vi "[RT]Intellirupter_Read.vi"() -> ()   [LabVIEW 2016]
uses:
  <vilib>/rvi/interface/nirviOpenFPGA/nirviOpenFPGA.xnode
  <vilib>/rvi/interface/nirviCloseFPGA/nirviCloseFPGA.xnode
  <vilib>/rvi/interface/nirviMethod/nirviMethod.xnode
  <vilib>/rvi/interface/nirviReadWriteControl/nirviReadWriteControl.xnode
  <vilib>/FPGAPlugInAG/Dynamic/niLvFpga_ReadFifo_Dynamic.vi
  <vilib>/rvi/errors/niLvFpgaMergeErrorWithErrorCode.vi
  FPGA Bitfiles/IntelliRupter_FPGATarget_Intelliruptersensor5.lvbitx
  <vilib>/FPGAPlugInAG/cRIO-9039 (Sync)/niLvFpga_Open_cRIO-9039 (Sync).vi
  <vilib>/rvi/interface/common/dynamic/niFpgaDynamicAddResources.vi
  <vilib>/rvi/interface/Simulation/niFpgaSimulationCallBeginRW.vi
  <vilib>/rvi/errors/niLvFpgaAdjustHostInterfaceError.vi
  <vilib>/FPGAPlugInAG/Dynamic/niLvFpga_Close_Dynamic.vi
panel:
  in  "Count(ticks)":u32
  out "Waveform Chart":dbl(graph)
  out "error out":errorcluster
  in  "Relay 2":bool
  in  "Relay 1":bool
  in  "Relay 4":bool
  in  "Relay 3":bool
  in  "Relay 5":bool
  in  "Relay 6":bool
  in  "Relay 8":bool
  in  "Relay 7":bool
  in  "Stop":bool
  out "I8 B":fxp<+/-,26,5>
  out "I8 A":fxp<+/-,26,5>
  out "V8R CA":fxp<+/-,26,5>
  out "V8R BC":fxp<+/-,26,5>
  out "V8R AB":fxp<+/-,26,5>
  out "V5R CA":fxp<+/-,26,5>
  out "V5R BC":fxp<+/-,26,5>
  out "V5R AB":fxp<+/-,26,5>
  out "I5 B":fxp<+/-,26,5>
  out "I5 A":fxp<+/-,26,5>
  out "V5L CA":fxp<+/-,26,5>
  out "V5L BC":fxp<+/-,26,5>
  out "V5L AB":fxp<+/-,26,5>
  out "V4L CA":fxp<+/-,26,5>
  out "V4L BC":fxp<+/-,26,5>
  out "V4L AB":fxp<+/-,26,5>
  out "I4 C":fxp<+/-,26,5>
  out "I4 B":fxp<+/-,26,5>
  out "I4 A":fxp<+/-,26,5>
  out "V4R CA":fxp<+/-,26,5>
  out "V4R BC":fxp<+/-,26,5>
  out "V4R AB":fxp<+/-,26,5>
  out "V2L CA":fxp<+/-,26,5>
  out "V2L BC":fxp<+/-,26,5>
  out "V2L AB":fxp<+/-,26,5>
  out "I2 C":fxp<+/-,26,5>
  out "I5 C":fxp<+/-,26,5>
  out "I2 B":fxp<+/-,26,5>
  out "I2 A":fxp<+/-,26,5>
  out "V2R CA":fxp<+/-,26,5>
  out "V2R BC":fxp<+/-,26,5>
  out "V2R AB":fxp<+/-,26,5>
  out "V7R CA":fxp<+/-,26,5>
  out "V7R BC":fxp<+/-,26,5>
  out "V7R AB":fxp<+/-,26,5>
  out "I8 C":fxp<+/-,26,5>
  out "V8L CA":fxp<+/-,26,5>
  out "V8L BC":fxp<+/-,26,5>
  out "V8L AB":fxp<+/-,26,5>
  out "I7 C":fxp<+/-,26,5>
  out "I7 B":fxp<+/-,26,5>
  out "I7 A":fxp<+/-,26,5>
  out "V7L CA":fxp<+/-,26,5>
  out "V7L BC":fxp<+/-,26,5>
  out "V7L AB":fxp<+/-,26,5>
  out "V6R CA":fxp<+/-,26,5>
  out "V6R BC":fxp<+/-,26,5>
  out "V6R AB":fxp<+/-,26,5>
  out "I6 C":fxp<+/-,26,5>
  out "I6 B":fxp<+/-,26,5>
  out "I6 A":fxp<+/-,26,5>
  out "V6L CA":fxp<+/-,26,5>
  out "V6L BC":fxp<+/-,26,5>
  out "V6L AB":fxp<+/-,26,5>
  out "V3L CA":fxp<+/-,26,5>
  out "V3L BC":fxp<+/-,26,5>
  out "V3L AB":fxp<+/-,26,5>
  out "I3 C":fxp<+/-,26,5>
  out "I3 B":fxp<+/-,26,5>
  out "I3 A":fxp<+/-,26,5>
  out "V3R CA":fxp<+/-,26,5>
  out "V3R BC":fxp<+/-,26,5>
  out "V3R AB":fxp<+/-,26,5>
  out "V1L CA":fxp<+/-,26,5>
  out "V1L BC":fxp<+/-,26,5>
  out "V1L AB":fxp<+/-,26,5>
  out "I1 C":fxp<+/-,26,5>
  out "I1 B":fxp<+/-,26,5>
  out "I1 A":fxp<+/-,26,5>
  out "V1R CA":fxp<+/-,12,5>
  out "V1R BC":fxp<+/-,26,5>
  out "V1R AB":fxp<+/-,26,5>
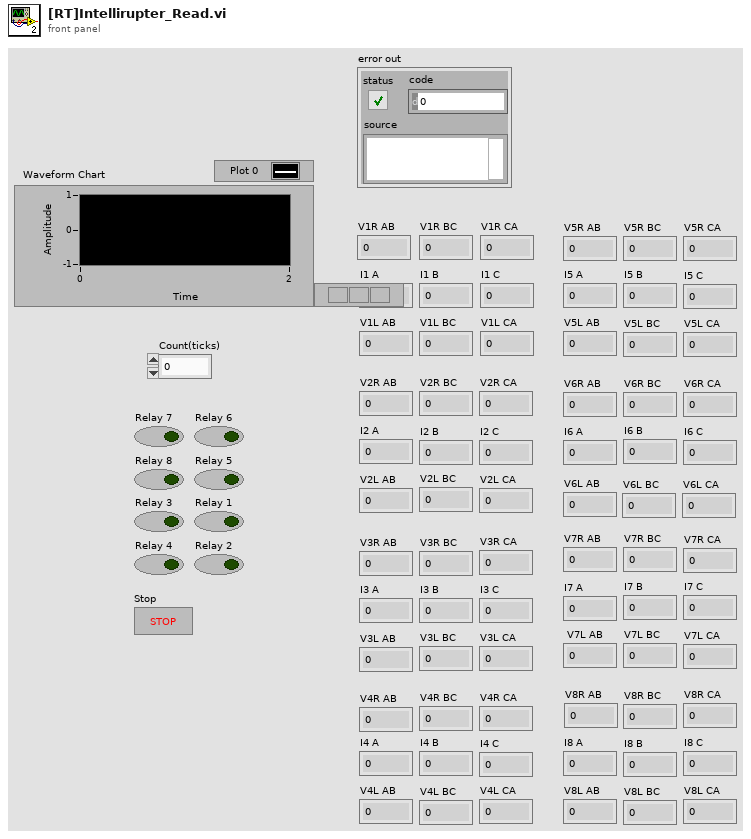
[diagram p1: front panel]
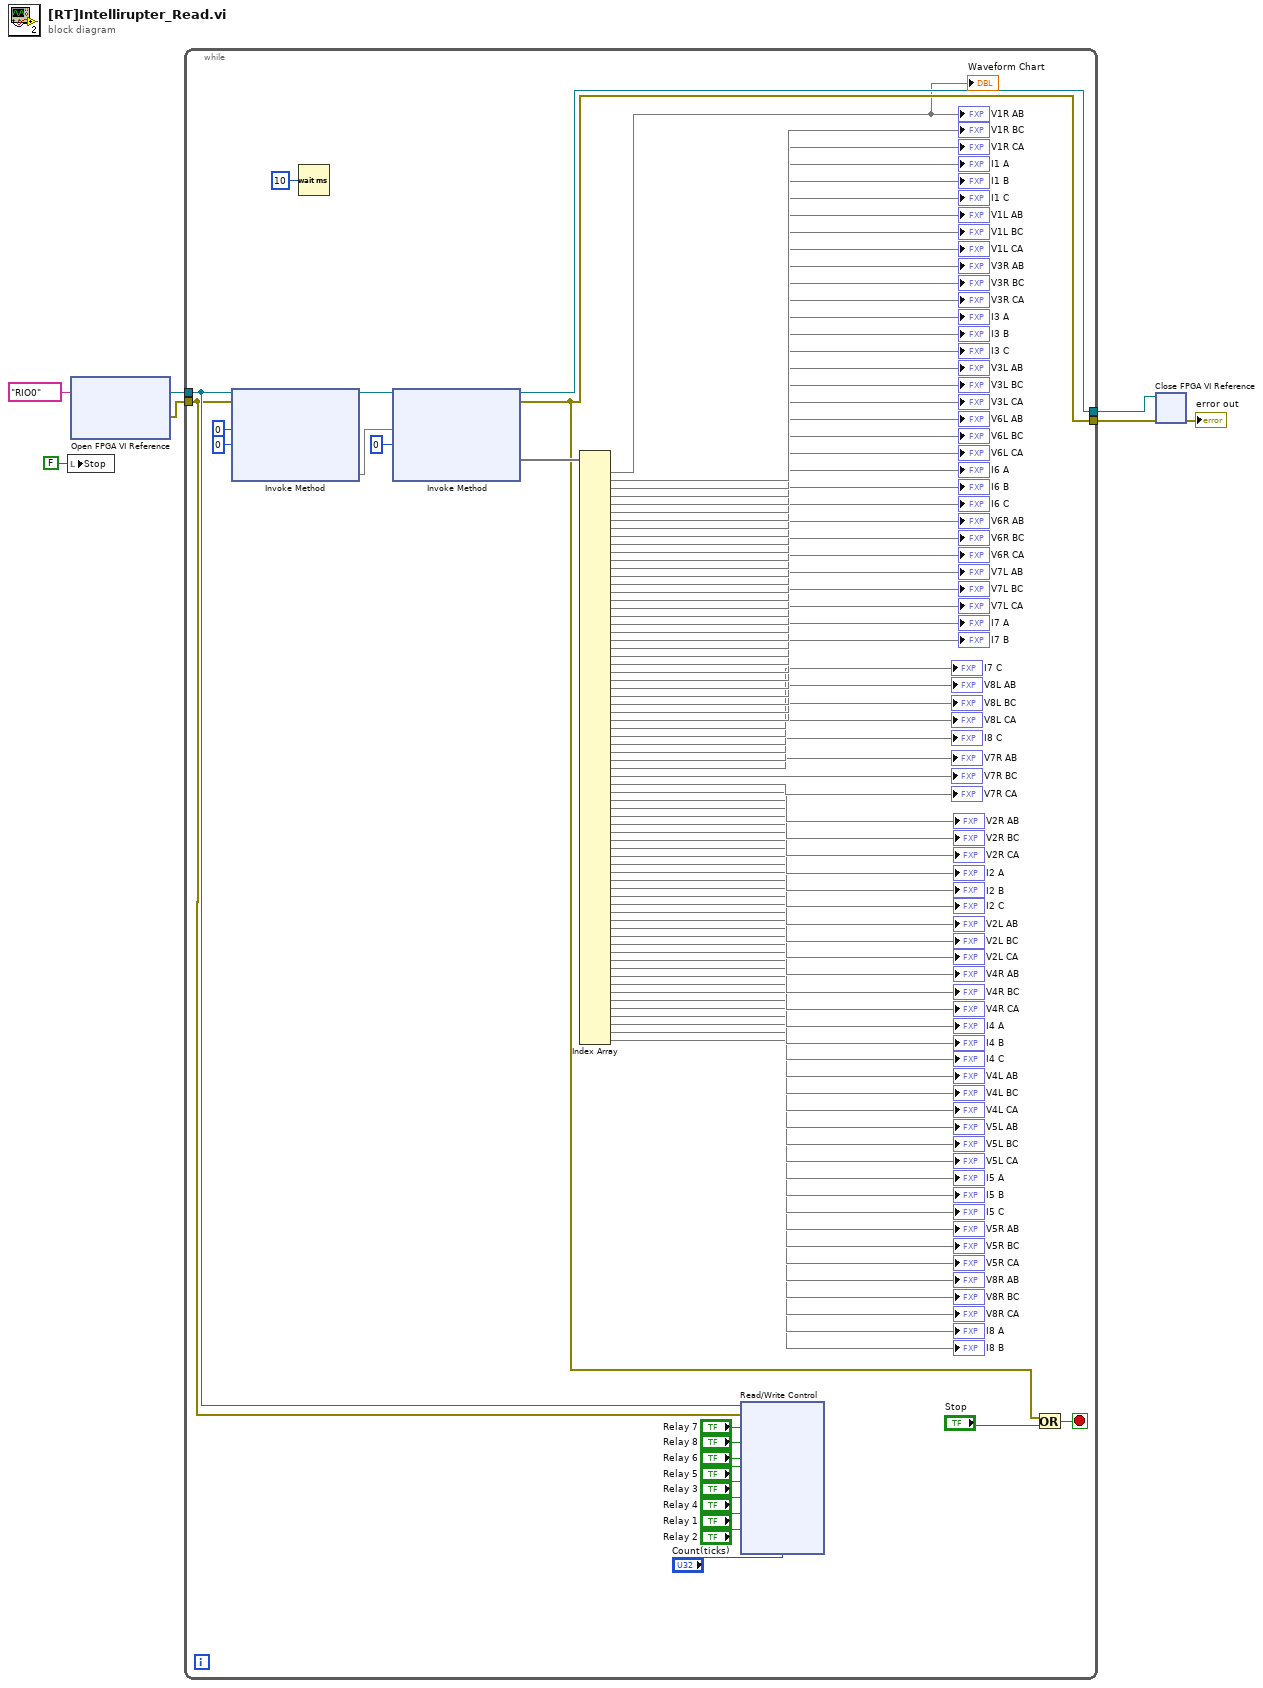
[diagram p0: block diagram]
diagram:
  n1 = local write "Stop"(FALSE ("Stop")) -> ()
  n2 = xnode "Open FPGA VI Reference"("resource name"=tag "RIO0") -> ("FPGA VI Reference Out"=w7:refnum<k20>, "error out"=w6:errorcluster)  [unwired: 1 in]
  n3 = while {
    tunnel: w7 -> [w25]
    tunnel: w6 -> [w24]
    tunnel: [w14] -> w5
    tunnel: [w10] -> w4
    stop <- w30 stop-if-true
    n4 = xnode "Invoke Method"("FPGA VI Reference In"=w25, "error in"=w24, "Number of Elements"=u32 0, "Timeout (ms)"=0) -> ("FPGA VI Reference Out"=w28:refnum<k20>, "Elements Remaining"=w12)  [unwired: 2 out]
    n5 = Wait (ms)(milliseconds to wait=u32 10) -> ()  [unwired: 1 out]
    n6 = xnode "Invoke Method"("FPGA VI Reference In"=w28, "Number of Elements"=w12, "Timeout (ms)"=0) -> ("FPGA VI Reference Out"=w14:refnum<k20>, "error out"=w10:errorcluster, "Data"=w11:void[])  [unwired: 1 in, 1 out]
    n7 = Index Array(array=w11) -> (element #1=→"V1R AB" →"Waveform Chart", element #2=→"V1R BC", element #3=→"V1R CA", element #4=→"I1 A", element #5=→"I1 B", element #6=→"I1 C", element #7=→"V1L AB", element #8=→"V1L BC", element #9=→"V1L CA", element #10=→"V3R AB", element #11=→"V3R BC", element #12=→"V3R CA", element #13=→"I3 A", element #14=→"I3 B", element #15=→"I3 C", element #16=→"V3L AB", element #17=→"V3L BC", element #18=→"V3L CA", element #19=→"V6L AB", element #20=→"V6L BC", element #21=→"V6L CA", element #22=→"I6 A", element #23=→"I6 B", element #24=→"I6 C", element #25=→"V6R AB", element #26=→"V6R BC", element #27=→"V6R CA", element #28=→"V7L AB", element #29=→"V7L BC", element #30=→"V7L CA", element #31=→"I7 A", element #32=→"I7 B", element #33=→"I7 C", element #34=→"V8L AB", element #35=→"V8L BC", element #36=→"V8L CA", element #37=→"I8 C", element #38=→"V7R AB", element #39=→"V7R BC", element #40=→"V7R CA", element #41=→"V2R AB", element #42=→"V2R BC", element #43=→"V2R CA", element #44=→"I2 A", element #45=→"I2 B", element #46=→"I2 C", element #47=→"V2L AB", element #48=→"V2L BC", element #49=→"V2L CA", element #50=→"V4R AB", element #51=→"V4R BC", element #52=→"V4R CA", element #53=→"I4 A", element #54=→"I4 B", element #55=→"I4 C", element #56=→"V4L AB", element #57=→"V4L BC", element #58=→"V4L CA", element #59=→"V5L AB", element #60=→"V5L BC", element #61=→"V5L CA", element #62=→"I5 A", element #63=→"I5 B", element #64=→"I5 C", element #65=→"V5R AB", element #66=→"V5R BC", element #67=→"V5R CA", element #68=→"V8R AB", element #69=→"V8R BC", element #70=→"V8R CA", element #71=→"I8 A", element #72=→"I8 B")  [unwired: 72 in]
    n8 = xnode "Read/Write Control"("FPGA VI Reference In"=w25, "error in"=w24, "Relay8"="Relay 7", "Relay7"="Relay 8", "Relay6"="Relay 6", "Relay5"="Relay 5", "Relay4"="Relay 3", "Relay3"="Relay 4", "Relay2"="Relay 1", "Relay1"="Relay 2", "Count(ticks)"="Count(ticks)") -> ()  [unwired: 2 out]
    n9 = Or(x=w10, y="Stop") -> (x .or. y?=w30:bool)
  }
  n10 = xnode "Close FPGA VI Reference"("FPGA VI Reference In"=w5, "error in"=w4) -> ("error out"=→"error out":errorcluster)
